vi "Filter50s s p 50.vi"(11 "u":dbl) -> (3 "y":dbl)   [LabVIEW 2018]
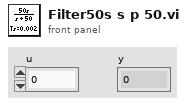
[diagram p1: front panel]
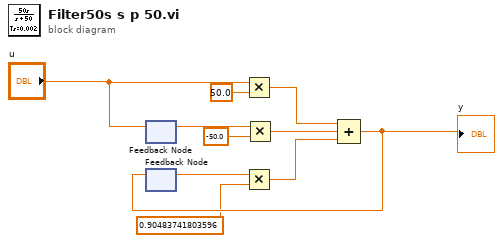
[diagram p0: block diagram]
diagram:
  n1 = feedback #1() -> (w3:dbl)  [unwired: 1 in]
  n2 = feedback-in #1 ("2")("u") -> ()
  n3 = feedback #2 ("Feedback Node 2")() -> (w6:dbl)  [unwired: 1 in]
  n4 = Multiply(x="u", y=50.0) -> (x*y=w8:dbl)
  n5 = Multiply ("Multiply 3")(x=w6, y=0.90483741803596 ("y 3")) -> (x*y=w9:dbl)
  n6 = Multiply ("Multiply 2")(x=w3, y=-50.0 ("y 2")) -> (x*y=w7:dbl)
  n7 = Compound Arithmetic op=ADD(w8, w7, w9) -> (w10:dbl)
  "y" <- w10
  n8 = feedback-in #2 ("3")(w10) -> ()
